vi "Get Plugin UI.vi"(8 "error in (no error)":errorcluster, 11 "Component UI in":refnum<class "RDMA User Interfaces.lvclass">) -> (0 "error out":errorcluster, 2 "Plugin Settings UI":refnum<class "User Interface.lvclass">, 3 "Component UI out":refnum<class "RDMA User Interfaces.lvclass">)   [LabVIEW 2020, in "RDMA.lvlib" / "RDMA User Interfaces.lvclass"]
uses:
  RDMA User Interfaces.lvclass
  DSF Core.lvlibp/Classes/User Interface/User Interface.lvclass
  Plugin/RDMA Plugin User Interface.lvclass
  C:/git/fmussi-niveristand-data-sharing-framework-custom-device-plugins/Components/DSF Core.lvlibp/Classes/User Interface/User Interface.lvclass
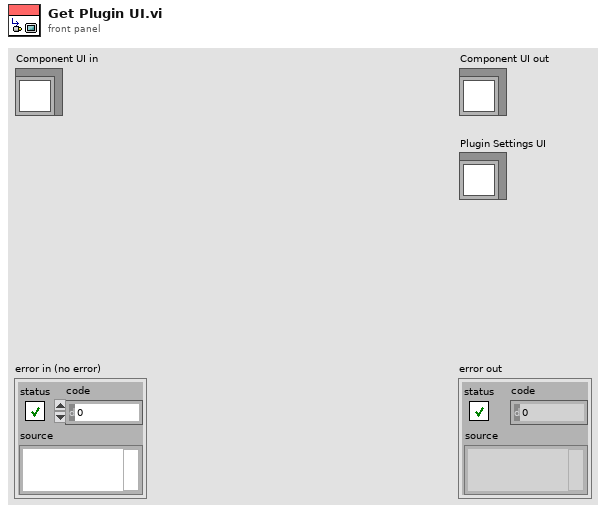
[diagram p1: front panel]
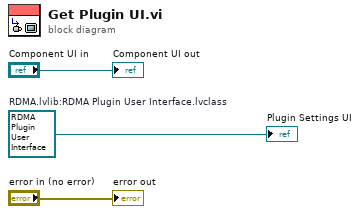
[diagram p0: block diagram]
diagram:
  w1 = refnum<class "RDMA Plugin User Interface.lvclass"> refnum  # RDMA.lvlib:RDMA Plugin User Interface.lvclass
  "error out" <- "error in (no error)"
  "Component UI out" <- "Component UI in"
  "Plugin Settings UI" <- w1
